vi "CallGenerator.vi"   [LabVIEW 2017]
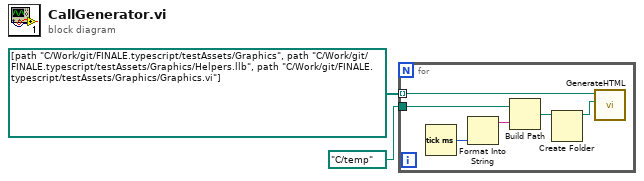
[diagram p0: block diagram]
diagram:
  n1 = for {
    tunnel: path[] [path "C:/Work/git/FINALE.typescript/testAssets/Graphics", path "C:/Work/git/FINALE.typescript/testAssets/Graphics/Helpers.llb", path "C:/Work/git/FINALE.typescript/testAssets/Graphics/Graphics.vi"] -> [w8] mode=indexing
    tunnel: path "C:/temp" -> [w7]
    n2 = Tick Count (ms)() -> (millisecond timer value=w6:u32)
    n3 = Format Into String(w6) -> (resulting string=w5:string)  [unwired: 3 in, 1 out]
    n4 = Build Path(base path=w7, name or relative path=w5) -> (appended path=w4:path)
    n5 = Create Folder(path (use dialog)=w4) -> (created path=w3:path)  [unwired: 2 in, 2 out]
    n6 = call "GenerateHTML.vi"("Destination Directory"=w3, "Source directory/files"=w8) -> ()  [unwired: 8 in, 2 out]
  }
